vi "InitDev.vi"(1 "SAVE?":bool, 2 "IP地址":string="192.168.1.16", 3 "SampleRate":T2(ring)=enum."105.468", 4 "SavePath":path) -> (0 "输出簇":T1)   [LabVIEW 2012]
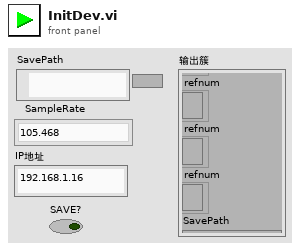
[diagram p1: front panel]
types:
  T1 = cluster{"refnum":refnum<file>, "refnum":refnum<file>, "refnum":refnum<file>, "refnum":refnum<file>, "refnum":refnum<file>, "SavePath":path, "SAVE?":bool, "connection ID":refnum<k5>}
  T2 = enum16{"", "105.468", "52.734", "35.156", "26.367", "21.094", "17.578", "15.067", "13.184", "11.719", "10.545"}
  T3 = enum16{"open", "replace", "create", "open or create", "replace or create", "replace or create with confirmation"}
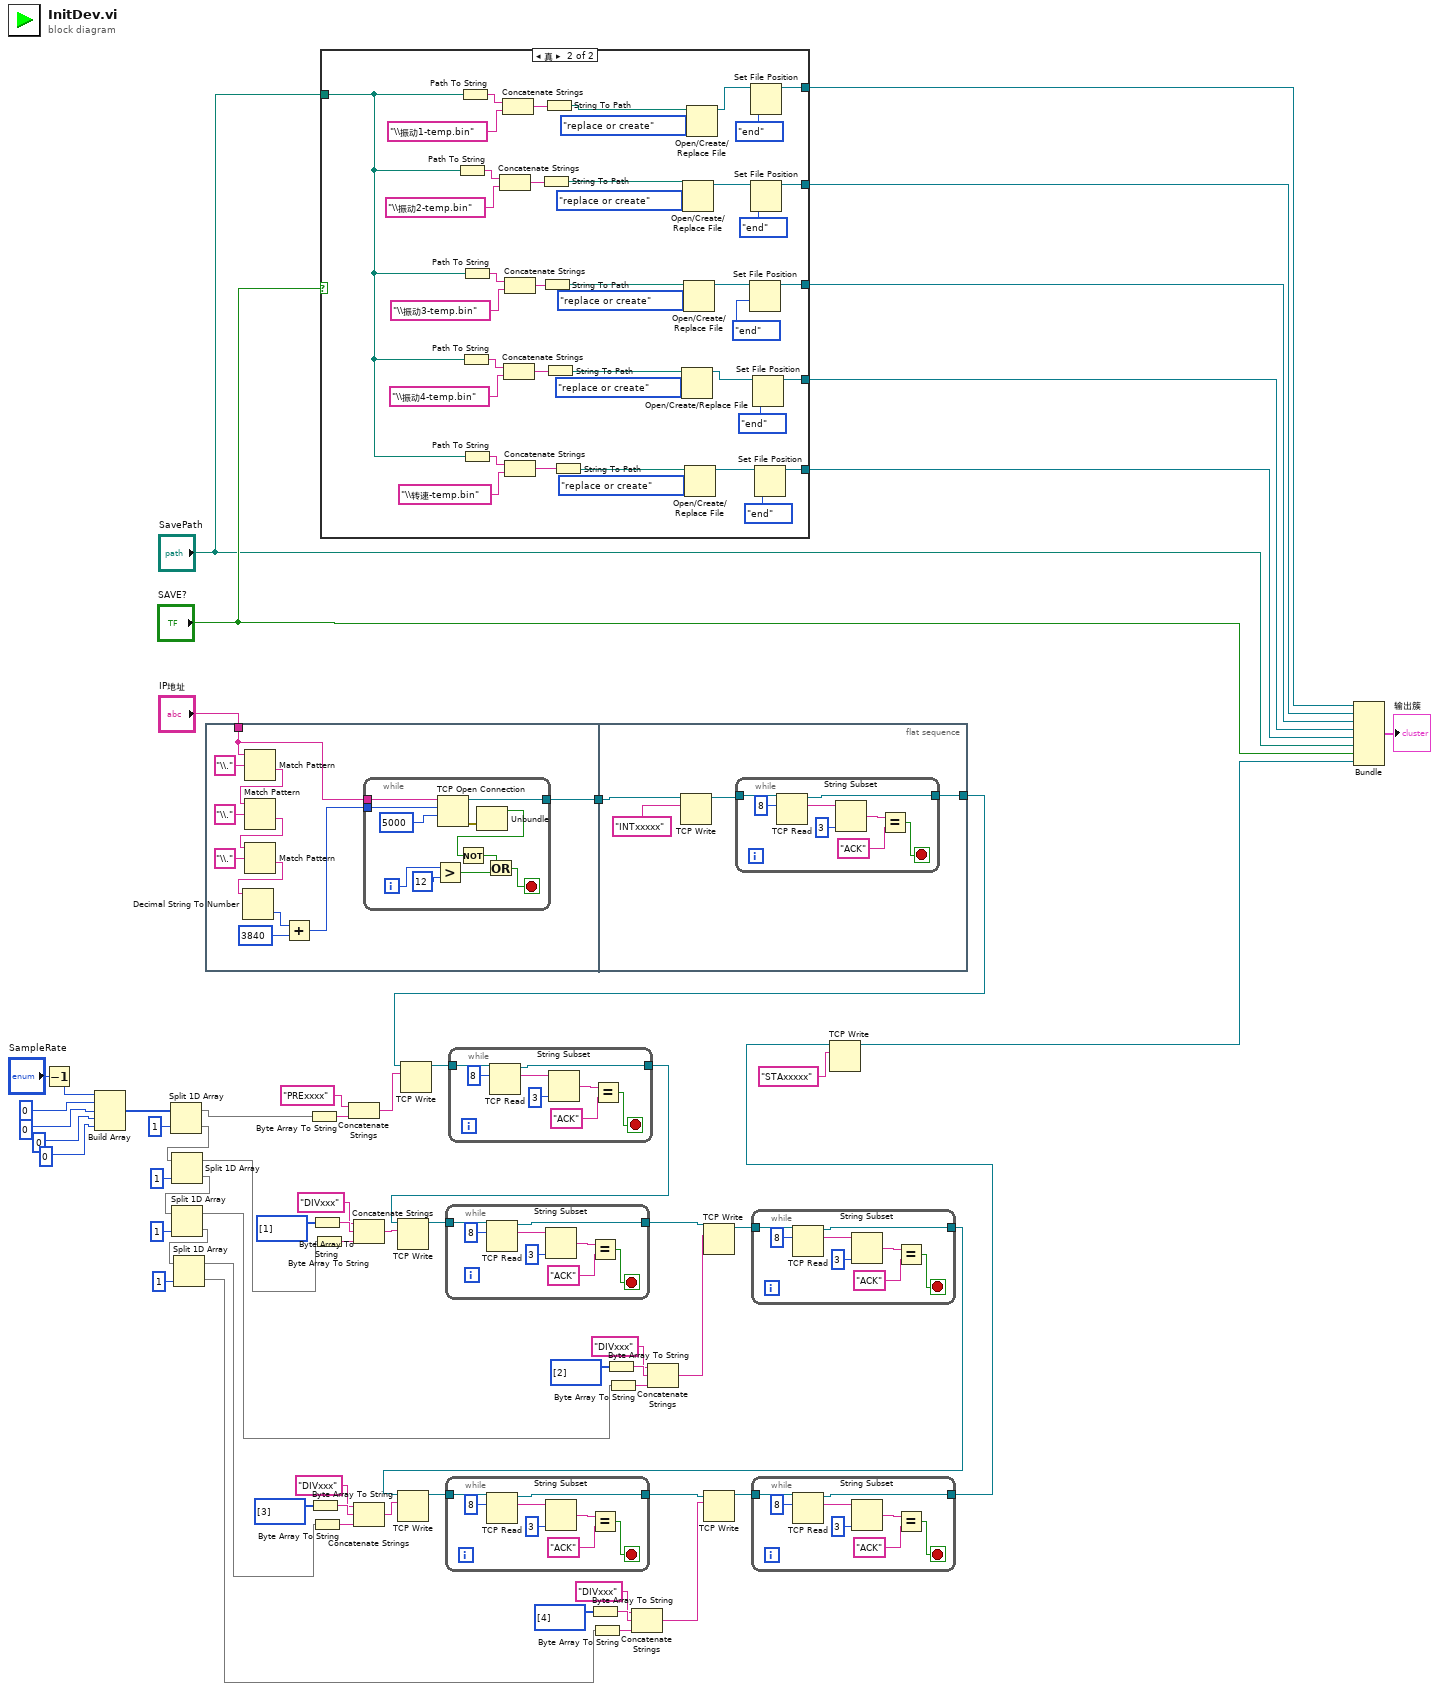
[diagram p0: block diagram]
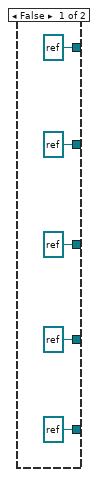
[diagram p2: hidden frame]
diagram:
  n1 = Decrement(x="SampleRate") -> (x-1=w10:T2)
  n2 = Build Array(w10, u8 0 ("元素"), u8 0 ("元素"), u8 0 ("元素"), u8 0 ("元素")) -> (w65:u16[])
  n3 = Split 1D Array(array=w65, index=1 ("索引")) -> (first subarray=w46:u16[], second subarray=w42:u16[])
  n4 = Split 1D Array(array=w42, index=1 ("索引")) -> (first subarray=w22:u16[], second subarray=w41:u16[])
  n5 = Split 1D Array(array=w41, index=1 ("索引")) -> (first subarray=w21:u16[], second subarray=w40:u16[])
  n6 = Split 1D Array(array=w40, index=1 ("索引")) -> (first subarray=w20:u16[], second subarray=w19:u16[])
  n7 = flat-sequence {
    tunnel: "IP地址" -> [w68]
    tunnel: [w66] -> w1
    tunnel: [w88] -> w13
    tunnel: w1 -> [w90]
    frame #0 {
      n8 = Match Pattern(string=w68, regular expression="\\." ("正则表达式")) -> (after substring=w72:string)  [unwired: 1 in, 3 out]
      n9 = Match Pattern(string=w72, regular expression="\\." ("正则表达式")) -> (after substring=w73:string)  [unwired: 1 in, 3 out]
      n10 = Match Pattern(string=w73, regular expression="\\." ("正则表达式")) -> (after substring=w74:string)  [unwired: 1 in, 3 out]
      n11 = Decimal String To Number(string=w74) -> (number=w75:i32)  [unwired: 2 in, 1 out]
      n12 = Add(x=w75, y=3840) -> (x+y=w67:i32)
      n13 = while {
        tunnel: w68 -> [w87]
        tunnel: w67 -> [w86]
        tunnel: [w85] -> w66
        i -> [w82]
        stop <- w79 stop-if-true
        n14 = Greater?(x=w82, y=12) -> (0:w80:bool)
        n15 = TCP Open Connection(address=w87, remote port or service name=w86, timeout ms (60000)=5000 ("超时毫秒(60000)")) -> (connection ID=w85:refnum<k5>, error out=w83:errorcluster)  [unwired: 2 in]
        n16 = Unbundle(w83) -> ("status"=w77:bool)  [unwired: 2 out]
        n17 = Not(x=w77) -> (.not. x?=w78:bool)
        n18 = Or(x=w78, y=w80) -> (x .or. y?=w79:bool)
      }
    }
    frame #1 {
      n19 = TCP Write(connection ID=w90, data in="INTxxxxx" ("数据输入")) -> (connection ID out=w89:refnum<k5>)  [unwired: 2 in, 2 out]
      n20 = while {
        tunnel: w89 -> [w99]
        tunnel: [w93] -> w88
        stop <- w94 stop-if-true
        n21 = TCP Read(connection ID=w99, bytes to read=8 ("读取的字节")) -> (connection ID out=w93:refnum<k5>, data out=w97:string)  [unwired: 3 in, 1 out]
        n22 = String Subset(string=w97, length (rest)=3 ("偏移量(0)")) -> (substring=w96:string)  [unwired: 1 in]
        n23 = Equal?(x=w96, y="ACK") -> (x = y?=w94:bool)
      }
    }
  }
  n24 = Byte Array To String(unsigned byte array=w46) -> (string=w50:string)
  n25 = Byte Array To String(unsigned byte array=u8[] [3] ("无符号字节数组")) -> (string=w28:string)
  n26 = Byte Array To String(unsigned byte array=u8[] [1] ("无符号字节数组")) -> (string=w36:string)
  n27 = Byte Array To String(unsigned byte array=w20) -> (string=w30:string)
  n28 = Byte Array To String(unsigned byte array=w22) -> (string=w39:string)
  n29 = case shown="真" "SAVE?" {
    tunnel: [refnum<file> refnum ("refnum") w125] -> w9
    tunnel: [refnum<file> refnum ("refnum") w124] -> w8
    tunnel: [refnum<file> refnum ("refnum") w123] -> w7
    tunnel: [refnum<file> refnum ("refnum") w122] -> w6
    tunnel: [refnum<file> refnum ("refnum") w121] -> w5
    tunnel: "SavePath" -> [_ w105]
    frame False {
    }
    frame True {
      n30 = Path To String(path=w105) -> (string=w119:string)
      n31 = Path To String(path=w105) -> (string=w120:string)
      n32 = Path To String(path=w105) -> (string=w117:string)
      n33 = Path To String(path=w105) -> (string=w118:string)
      n34 = Path To String(path=w105) -> (string=w116:string)
      n35 = Concatenate Strings(w119, "\\振动2-temp.bin" ("字符串")) -> (w109:string)
      n36 = Concatenate Strings(w120, "\\振动1-temp.bin" ("字符串")) -> (w110:string)
      n37 = Concatenate Strings(w117, "\\振动4-temp.bin" ("字符串")) -> (w107:string)
      n38 = Concatenate Strings(w118, "\\振动3-temp.bin" ("字符串")) -> (w108:string)
      n39 = Concatenate Strings(w116, "\\转速-temp.bin" ("字符串")) -> (w106:string)
      n40 = String To Path(string=w109) -> (path=w134:path)
      n41 = String To Path(string=w108) -> (path=w133:path)
      n42 = String To Path(string=w110) -> (path=w135:path)
      n43 = String To Path(string=w107) -> (path=w132:path)
      n44 = String To Path(string=w106) -> (path=w131:path)
      n45 = Open/Create/Replace File(file path (use dialog)=w132, operation (0:open)=T3."replace or create" ("操作(0:open)")) -> (refnum out=w142:refnum<file>)  [unwired: 4 in, 2 out]
      n46 = Open/Create/Replace File(file path (use dialog)=w134, operation (0:open)=T3."replace or create" ("操作(0:open)")) -> (refnum out=w144:refnum<file>)  [unwired: 4 in, 2 out]
      n47 = Open/Create/Replace File(file path (use dialog)=w133, operation (0:open)=T3."replace or create" ("操作(0:open)")) -> (refnum out=w143:refnum<file>)  [unwired: 4 in, 2 out]
      n48 = Open/Create/Replace File(file path (use dialog)=w131, operation (0:open)=T3."replace or create" ("操作(0:open)")) -> (refnum out=w141:refnum<file>)  [unwired: 4 in, 2 out]
      n49 = Open/Create/Replace File(file path (use dialog)=w135, operation (0:open)=T3."replace or create" ("操作(0:open)")) -> (refnum out=w145:refnum<file>)  [unwired: 4 in, 2 out]
      n50 = Set File Position(refnum=w143, from (0:start)=enum16{"start", "end", "current"}."end" ("自（0:起始）")) -> (refnum out=w123:refnum<file>)  [unwired: 2 in, 1 out]
      n51 = Set File Position(refnum=w145, from (0:start)=enum16{"start", "end", "current"}."end" ("自（0:起始）")) -> (refnum out=w125:refnum<file>)  [unwired: 2 in, 1 out]
      n52 = Set File Position(refnum=w144, from (0:start)=enum16{"start", "end", "current"}."end" ("自（0:起始）")) -> (refnum out=w124:refnum<file>)  [unwired: 2 in, 1 out]
      n53 = Set File Position(refnum=w142, from (0:start)=enum16{"start", "end", "current"}."end" ("自（0:起始）")) -> (refnum out=w122:refnum<file>)  [unwired: 2 in, 1 out]
      n54 = Set File Position(refnum=w141, from (0:start)=enum16{"start", "end", "current"}."end" ("自（0:起始）")) -> (refnum out=w121:refnum<file>)  [unwired: 2 in, 1 out]
    }
  }
  n55 = Concatenate Strings("PRExxxx" ("数据输入"), w50) -> (w48:string)
  n56 = Concatenate Strings("DIVxxx" ("数据输入"), w36, w39) -> (w38:string)
  n57 = Concatenate Strings("DIVxxx" ("数据输入"), w28, w30) -> (w14:string)
  n58 = TCP Write(connection ID=w13, data in=w48) -> (connection ID out=w59:refnum<k5>)  [unwired: 2 in, 2 out]
  n59 = while {
    tunnel: w59 -> [w153]
    tunnel: [w147] -> w54
    stop <- w148 stop-if-true
    n60 = TCP Read(connection ID=w153, bytes to read=8 ("读取的字节")) -> (connection ID out=w147:refnum<k5>, data out=w151:string)  [unwired: 3 in, 1 out]
    n61 = String Subset(string=w151, length (rest)=3 ("偏移量(0)")) -> (substring=w150:string)  [unwired: 1 in]
    n62 = Equal?(x=w150, y="ACK") -> (x = y?=w148:bool)
  }
  n63 = TCP Write(connection ID=w54, data in=w38) -> (connection ID out=w58:refnum<k5>)  [unwired: 2 in, 2 out]
  n64 = while {
    tunnel: w58 -> [w161]
    tunnel: [w155] -> w53
    stop <- w156 stop-if-true
    n65 = TCP Read(connection ID=w161, bytes to read=8 ("读取的字节")) -> (connection ID out=w155:refnum<k5>, data out=w159:string)  [unwired: 3 in, 1 out]
    n66 = String Subset(string=w159, length (rest)=3 ("偏移量(0)")) -> (substring=w158:string)  [unwired: 1 in]
    n67 = Equal?(x=w158, y="ACK") -> (x = y?=w156:bool)
  }
  n68 = Byte Array To String(unsigned byte array=u8[] [4] ("无符号字节数组")) -> (string=w24:string)
  n69 = Byte Array To String(unsigned byte array=w19) -> (string=w26:string)
  n70 = Byte Array To String(unsigned byte array=u8[] [2] ("无符号字节数组")) -> (string=w32:string)
  n71 = Byte Array To String(unsigned byte array=w21) -> (string=w34:string)
  n72 = Concatenate Strings("DIVxxx" ("数据输入"), w24, w26) -> (w17:string)
  n73 = Concatenate Strings("DIVxxx" ("数据输入"), w32, w34) -> (w18:string)
  n74 = TCP Write(connection ID=w53, data in=w18) -> (connection ID out=w57:refnum<k5>)  [unwired: 2 in, 2 out]
  n75 = while {
    tunnel: w57 -> [w169]
    tunnel: [w163] -> w52
    stop <- w164 stop-if-true
    n76 = TCP Read(connection ID=w169, bytes to read=8 ("读取的字节")) -> (connection ID out=w163:refnum<k5>, data out=w167:string)  [unwired: 3 in, 1 out]
    n77 = String Subset(string=w167, length (rest)=3 ("偏移量(0)")) -> (substring=w166:string)  [unwired: 1 in]
    n78 = Equal?(x=w166, y="ACK") -> (x = y?=w164:bool)
  }
  n79 = TCP Write(connection ID=w52, data in=w14) -> (connection ID out=w56:refnum<k5>)  [unwired: 2 in, 2 out]
  n80 = while {
    tunnel: w56 -> [w177]
    tunnel: [w171] -> w51
    stop <- w172 stop-if-true
    n81 = TCP Read(connection ID=w177, bytes to read=8 ("读取的字节")) -> (connection ID out=w171:refnum<k5>, data out=w175:string)  [unwired: 3 in, 1 out]
    n82 = String Subset(string=w175, length (rest)=3 ("偏移量(0)")) -> (substring=w174:string)  [unwired: 1 in]
    n83 = Equal?(x=w174, y="ACK") -> (x = y?=w172:bool)
  }
  n84 = TCP Write(connection ID=w51, data in=w17) -> (connection ID out=w55:refnum<k5>)  [unwired: 2 in, 2 out]
  n85 = while {
    tunnel: w55 -> [w185]
    tunnel: [w179] -> w16
    stop <- w180 stop-if-true
    n86 = TCP Read(connection ID=w185, bytes to read=8 ("读取的字节")) -> (connection ID out=w179:refnum<k5>, data out=w183:string)  [unwired: 3 in, 1 out]
    n87 = String Subset(string=w183, length (rest)=3 ("偏移量(0)")) -> (substring=w182:string)  [unwired: 1 in]
    n88 = Equal?(x=w182, y="ACK") -> (x = y?=w180:bool)
  }
  n89 = TCP Write(connection ID=w16, data in="STAxxxxx" ("数据输入")) -> (connection ID out=w12:refnum<k5>)  [unwired: 2 in, 2 out]
  n90 = Bundle("refnum"=w9, "refnum"=w8, "refnum"=w7, "refnum"=w6, "refnum"=w5, "SavePath"="SavePath", "SAVE?"="SAVE?", "connection ID"=w12) -> (→"输出簇":T1)  [unwired: 1 in]
